vi "FPGA PPS Output_IC3172.vi"() -> ()   [LabVIEW 2017]
uses:
  <vilib>/Platform/TimedLoop/XDataNode/timing_clust.ctl
  <vilib>/Platform/TimedLoop/XDataNode/nitl_modes.ctl
  <vilib>/Platform/TimedLoop/XDataNode/wakeup.ctl
  <vilib>/rvi/eio/common/nirviEmuTemplateMethod_errors.vi
  <vilib>/rvi/Emulation/niFpgaSctlEmulationGetInTimedLoop.vi
  <vilib>/rvi/Emulation/niFpgaEmulationReportErrorSimple.vi
  <vilib>/rvi/Emulation/niFpgaGetClockAttributes.vi
  <vilib>/rvi/Emulation/niFpgaCriticalErrorInLSC.vi
  <vilib>/Platform/TimedLoop/XDataNode/XDataNode.xnode
  <vilib>/eio/EIONode/EIONode.xnode
  <vilib>/Platform/TimedLoop/XDataNode/XDNodeRunTimeDep.lvlib
panel:
  out "Current Time(ns)":u64
  in  "PPS.Update":bool
  in  "PPS.Time (ns)":u64
  in  "PPS. Pulse duration (ns)":i32=10000 format="%.0p"
  out "PPS. Pulse":bool
  # "This outputs a pulse per second based on the absolute time on the FPGA.  Normally no host interaction is needed but if time jumps then the host can reset the absolute time by reading the current time on the host and writing the U64 value of the next second to the PPS.Time (ns) and setting the PPS.Update to true."
  # "PPS Settings"
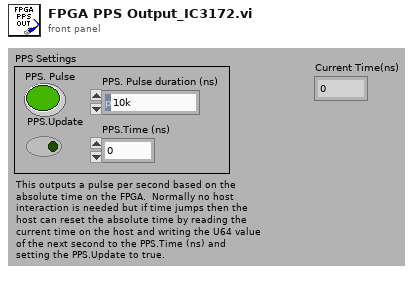
[diagram p1: front panel]
types:
  T1 = typedef "XDNodeRunTimeDep.lvlib/timing_clust.ctl" = cluster{"Expected End [f-1]":u64, "Actual End [f-1]":u64, "Finished Late? [f-1]":bool, "Expected End [i-1]":u64, "Actual End [i-1]":u64, "Finished Late? [i-1]":bool, "Expected Start [i]":u64, "Actual Start [i]":u64, "Expected Start [f]":u64, "Actual Start [f]":u64, "Source Name":string, "Structure Name":string, "Period":i64, "Deadline":i64, "Offset":i64, "Start":i64, "Priority":i32, "Timeout":i32, "Mode":T2, "Wakeup Reason":T3, "Error":errorcluster, "Source Type":string, "Secondary Source Type":string, "Global End Time":u64, "Global Start Time":u64, "Frame Duration":u64, "Iteration Duration":u64, "Assigned CPU":i32, "I/O Scan Engine Mode":u32}
  T2 = typedef "XDNodeRunTimeDep.lvlib/nitl_modes.ctl" = enum32{"No Change", "Process missed periods, maintain original phase", "Discard missed periods, maintain original phase", "Process missed periods, ignore original phase", "Discard missed periods, ignore original phase"}
  T3 = typedef "XDNodeRunTimeDep.lvlib/wakeup.ctl" = enum32{"Normal", "Aborted", "Asynchronous wakeup", "Timing source error", "Timed loop error", "Timeout"}
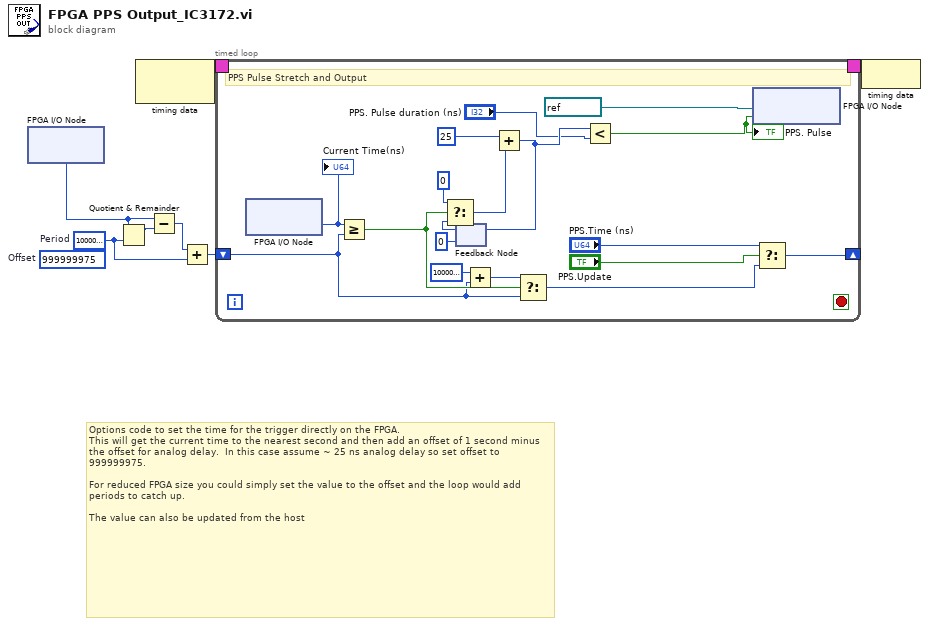
[diagram p0: block diagram]
diagram:
  (unwired) 999999975  # Offset
  w1 = u32 1000000000  # Period
  # "Options code to set the time for the trigger directly on the FPGA.\nThis will get the current time to the nearest second and then add an offset of 1 second minus the offset for analog delay.  In this case assume ~ 25 ns analog delay so set offset to 999999975.\n\nFor reduced FPGA size you could simply set the value to the offset and the loop would add periods to catch up. \n\nThe value can also be updated from the host"
  n1 = xnode "FPGA I/O Node"() -> ("Time"=w2:u64)  [unwired: 1 in, 1 out]
  n2 = Quotient & Remainder(x=w2, y=w1) -> (x-y*floor(x/y)=w5:u64)  [unwired: 1 out]
  n3 = node-c288() -> (w7:T1)  [unwired: 1 in]
  n4 = Subtract(x=w2, y=w5) -> (x-y=w4:u64)
  n5 = Add(x=w4, y=w1) -> (x+y=w3:u64)
  n6 = timed-loop {
    timing: w7 -> [_]
    timing-out: [_] -> w6
    shift-right: [w17] -> _
    shift-left: w3 -> [w16]
    stop <- _ stop-if-true
    # "PPS Pulse Stretch and Output"
    n7 = xnode "FPGA I/O Node"() -> ("Time"=w25:u64)  [unwired: 1 in, 1 out]
    "Current Time(ns)" <- w25
    n8 = Greater Or Equal?(x=w25, y=w16) -> (x >= y?=w19:bool)
    n9 = feedback #1(0) -> (w21:i32)
    n10 = Select(t=0, s=w19, f=w21) -> (s? t:f=w13:i32)
    n11 = Add(x=u32 1000000000 ("Period (ns)"), y=w16) -> (x+y=w24:u64)
    n12 = Add(x=25, y=w13) -> (x+y=w10:i32)
    n13 = feedback-in #1(w10) -> ()
    n14 = Select(t=w24, s=w19, f=w16) -> (s? t:f=w22:u64)
    n15 = Less?(x=w10, y="PPS. Pulse duration (ns)") -> (x < y?=w11:bool)
    "PPS. Pulse" <- w11
    n16 = xnode "FPGA I/O Node"("I/O Item"=w11, "FPGA I/O In"=refnum<k21> "TTL 0" ("PPS Output")) -> ()  [unwired: 1 out]
    n17 = Select(t="PPS.Time (ns)", s="PPS.Update", f=w22) -> (s? t:f=w17:u64)
  }
  n18 = node-c288(w6) -> ()
